vi "Launch Image Handler.vi"(8 "error in (no error)":errorcluster, 11 "Controller in":refnum<class "Controller.lvclass">) -> (0 "error out":errorcluster, 3 "Controller out":refnum<class "Controller.lvclass">)   [LabVIEW 2022 SP3, in "Controller.lvlib" / "Controller.lvclass"]
uses:
  Controller.lvclass
  C:/Program Files/National Instruments/LabVIEW 2022/vi.lib/ActorFramework/Actor/Actor.lvclass
  ImageHandler/ImageHandler/ImageHandler.lvclass
  Controller.lvclass/Controller.ctl
  UserInterface/UserInterface Messages/Log Data Msg/Log Data Msg.lvclass/Log Data Msg.ctl
  <vilib>/ActorFramework/Message Enqueuer/Message Enqueuer.lvclass/Message Enqueuer.ctl
  <vilib>/ActorFramework/Message Enqueuer/Enqueue.vi
  UserInterface/UserInterface Messages/Log Data Msg/Log Data Msg.lvclass
  C:/Program Files/National Instruments/LabVIEW 2022/vi.lib/ActorFramework/Message/Message.lvclass
  ImageHandler/ImageHandler Messages/Init Msg/Init Msg.lvclass
  <vilib>/ActorFramework/Message Priority Queue/Priority Enqueue.vi
  <vilib>/ActorFramework/Actor/Actor.lvclass
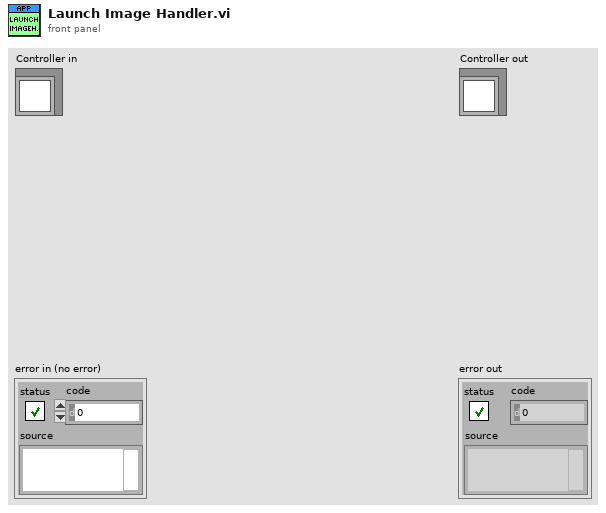
[diagram p1: front panel]
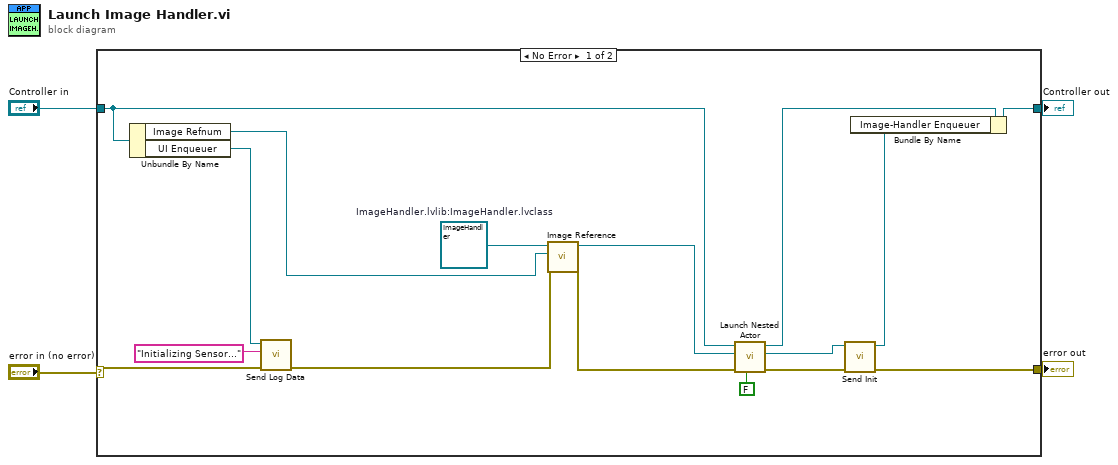
[diagram p0: block diagram]
diagram:
  n1 = case shown="No Error" "error in (no error)" {
    selector: "error in (no error)" -> [w13 w22]
    tunnel: [w11 w22] -> w3
    tunnel: [w16 w21] -> w1
    tunnel: "Controller in" -> [w15 w21]
    frame No Error {
      w19 = refnum<class "ImageHandler.lvclass"> refnum  # ImageHandler.lvlib:ImageHandler.lvclass
      n2 = Unbundle By Name(w15) -> ("Image Refnum"=w7:refnum<vi>, "UI Enqueuer"=w14:refnum<class "Message Enqueuer.lvclass">)
      n3 = call "Send Log Data.vi"("error in (no error)"=w13, "Message"="Initializing Sensor...", "Message Enqueuer"=w14) -> ("error out"=w6:errorcluster)  [unwired: 7 in, 1 out]
      n4 = call "Image Reference.vi"("error in (no error)"=w6, "Image Refnum"=w7, "ImageHandler in"=w19) -> ("error out"=w5:errorcluster, "ImageHandler out"=w8:refnum<class "ImageHandler.lvclass">)  [unwired: 7 in]
      n5 = call <vilib>:"Launch Nested Actor.vi"("Open Actor Core front panel? (F)"=FALSE, "error in (no error)"=w5, "Nested Actor"=w8, "Caller Actor in"=w15) -> ("error out"=w20:errorcluster, "Nested Actor's Enqueuer"=w10:refnum<class "Message Enqueuer.lvclass">, "Caller Actor out"=w17:refnum<class "Controller.lvclass">)  [unwired: 5 in]
      n6 = call "Send Init.vi"("error in (no error)"=w20, "Message Enqueuer"=w10) -> ("error out"=w11:errorcluster, "Message Enqueuer out"=w9:refnum<class "Message Enqueuer.lvclass">)  [unwired: 8 in]
      n7 = Bundle By Name(cluster=w17, "Image-Handler Enqueuer"=w9) -> (w16:refnum<class "Controller.lvclass">)
    }
    frame Error {
    }
  }
  "error out" <- w3
  "Controller out" <- w1
